vi "RegisterMat_Array2D-SGL.vi"(8 "error in":errorcluster, 11 "Array in":sgl[][](array[numeric])) -> (0 "error out":errorcluster, 3 "Image":u8, 4 "AdressOrData":sgl[][](array[numeric]), 6 "Mat":T1)   [LabVIEW 2020, in "OpenLvVision_OpenCv.lvlib"]
doc: "Register mat for dll.\nNo malleable to breake vi inlining!"
uses:
  OpenLvVision_OpenCv.lvlib
  TypeDef/MatInfo.ctl
  TypeDef/LvDatatype.ctl
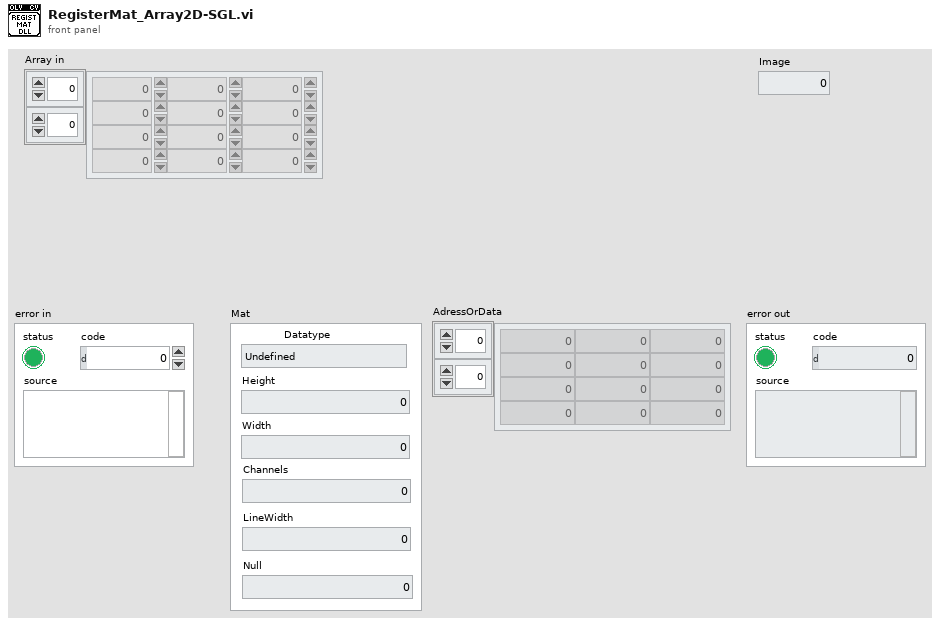
[diagram p1: front panel]
types:
  T1 = typedef "OpenLvVision_OpenCv.lvlib/MatInfo.ctl" = cluster{"Datatype":T2, "Height":i32, "Width":i32, "Channels":i32, "LineWidth":i32, "Null":u8}
  T2 = typedef "OpenLvVision_OpenCv.lvlib/LvDatatype.ctl" = enum32{"Undefined", "U8", "I8", "U16", "I16", "U32_Color", "I32", "U64_Color", "I64", "SGL", "DBL", "Complex SGL", "Complex DBL", "Array 1D U8", "Array 1D I8", "Array 1D U16", "Array 1D I16", "Array 1D U32_Color", "Array 1D I32", "Array 1D U64_Color", "Array 1D I64", "Array 1D SGL", "Array 1D DBL", "Array 1D Complex SGL", "Array 1D Complex DBL", "Array 2D U8", "Array 2D I8", "Array 2D U16", "Array 2D I16", "Array 2D U32", "Array 2D U32_Color", "Array 2D I32", "Array 2D U64", "Array 2D U64_Color", "Array 2D I64", "Array 2D SGL", "Array 2D DBL", "Array 2D Complex SGL", "Array 2D Complex DBL", "Image Mono U8", "Image Mono U16", "Image Mono I16", "Image Mono SGL", "Image Color U32", "Image Color U64", "ImageComplex Sgl"}
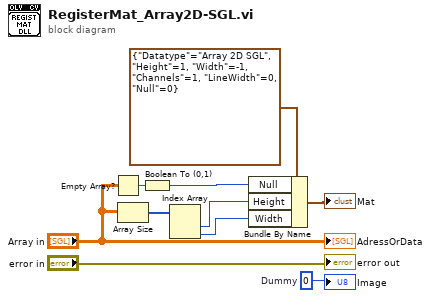
[diagram p0: block diagram]
diagram:
  w5 = u8 0  # Dummy
  n1 = Empty Array?(array="Array in") -> (empty?=w9:bool)
  n2 = Array Size(array="Array in") -> (size(s)=w3:i32[])
  n3 = Boolean To (0,1)(Boolean=w9) -> (0, 1=w8:i16)
  n4 = Index Array(array=w3) -> (element #1=w2:i32, element #2=w1:i32)  [unwired: 2 in]
  n5 = Bundle By Name(cluster=T1 {"Datatype"=enum."Array 2D SGL", "Height"=1, "Width"=-1, "Channels"=1, "LineWidth"=0, "Null"=0} ("LvData"), "Null"=w8, "Height"=w2, "Width"=w1) -> (→"Mat":T1)
  "error out" <- "error in"
  "AdressOrData" <- "Array in"
  "Image" <- w5
